vi "NStageMRate Decimation (Host).vi"(11 "multirate filters":T2[](array[typedef])=[{"mMRate_Structure"=enum."FIR", "mMRate_Mode"=2, "mMRate_Factor"=10, "mMRate_FIRParams"={"mMRate_FIR_H"=[0.00020851805806128276, 0.000613272420690698, 0.0014304185003561158, 0.0028435740310915566, 0.005060843192894627, 0.008276672977011198, 0.01263671879692099, 0.018200819196418323, 0.024910685996005263, 0.03256926849828543, 0.040837119060937545, 0.049249902078079846, 0.0572560861411628, 0.06427222716854132, 0.06974798706333393, 0.07323191327535455, 0.07442764407493105, 0.07323191327535455, 0.06974798706333393, 0.06427222716854132, 0.0572560861411628, 0.049249902078079846, 0.040837119060937545, 0.03256926849828543, 0.024910685996005263, 0.018200819196418323, 0.01263671879692099, 0.008276672977011198, 0.005060843192894627, 0.0028435740310915566, 0.0014304185003561158, 0.000613272420690698, 0.00020851805806128276], "mMRate_FIR_IsNyquist?"=FALSE, "mMRate_FIR_IsSymmetric?"=FALSE}, "mMRate_CICParams"={"mMRate_CIC_#Stage"=0, "mMRate_CIC_Lag"=0, "mMRate_CIC_Type"=enum."Lowpass"}, "mMRate_Order"=32, "mMRate_Version"="2.0", "mMRate_Comments"="", "mMRate_RationalFactor"={"mMRate_L"=-1, "mMRate_M"=-1}, "mMRate_Fs"=100000.0, "mMRate_Quantized?"=TRUE, "mMRate_QFilterGain"=1.0, "mMRate_CoefWl"=16, "mMRate_Scaling"={"mMRate_ScaleByPowerOf2?"=TRUE, "mMRate_ScaleType"=enum."Time Domain 1-Norm"}, "mMRate_InputWl"=16, "mMRate_OutputWl"=32, "mMRate_OutputMode"=enum."Nearest", "mMRate_MultMode"=enum."Truncated", "mMRate_BitPruning"=TRUE, "mMRate_GainWl"=-1, "mMRate_OutputFwl"=-30, "mMRate_SumIwl"=2, "mMRate_InputIwl "=1, "mMRate_SumWl"=32, "mMRate_CoefIwl"=0}, {"mMRate_Structure"=enum."FIR", "mMRate_Mode"=2, "mMRate_Factor"=5, "mMRate_FIRParams"={"mMRate_FIR_H"=[-0.0004681667078035737, -0.001767925193669993, -0.003970356160230413, -0.005978286856899856, -0.005090123043269885, 0.0025917170420743487, 0.020602728875030812, 0.04989465476912974, 0.08711166887294974, 0.12459826753370787, 0.15261700974431505, 0.1630150884241493, 0.15261700974431505, 0.12459826753370787, 0.08711166887294974, 0.04989465476912974, 0.020602728875030812, 0.0025917170420743487, -0.005090123043269885, -0.005978286856899856, -0.003970356160230413, -0.001767925193669993, -0.0004681667078035737], "mMRate_FIR_IsNyquist?"=FALSE, "mMRate_FIR_IsSymmetric?"=FALSE}, "mMRate_CICParams"={"mMRate_CIC_#Stage"=0, "mMRate_CIC_Lag"=0, "mMRate_CIC_Type"=enum."Lowpass"}, "mMRate_Order"=22, "mMRate_Version"="2.0", "mMRate_Comments"="", "mMRate_RationalFactor"={"mMRate_L"=-1, "mMRate_M"=-1}, "mMRate_Fs"=10000.0, "mMRate_Quantized?"=TRUE, "mMRate_QFilterGain"=2.0, "mMRate_CoefWl"=16, "mMRate_Scaling"={"mMRate_ScaleByPowerOf2?"=TRUE, "mMRate_ScaleType"=enum."Time Domain 1-Norm"}, "mMRate_InputWl"=32, "mMRate_OutputWl"=32, "mMRate_OutputMode"=enum."Nearest", "mMRate_MultMode"=enum."Truncated", "mMRate_BitPruning"=TRUE, "mMRate_GainWl"=-1, "mMRate_OutputFwl"=-30, "mMRate_SumIwl"=2, "mMRate_InputIwl "=1, "mMRate_SumWl"=32, "mMRate_CoefIwl"=0}, {"mMRate_Structure"=enum."FIR", "mMRate_Mode"=2, "mMRate_Factor"=2, "mMRate_FIRParams"={"mMRate_FIR_H"=[0.00011146621958819476, 0.0002565535621370625, 0.0004667088173512661, 0.0007398841585625596, 0.0009920839582570331, 0.0011689556532843148, 0.0011441466836693446, 0.0008511401604360608, 0.00021389293056072765, -0.0007249166118789748, -0.001870429374643854, -0.002986975146976202, -0.003801687060362348, -0.00398217847599286, -0.0032847785470121646, -0.0015737370213748415, 0.001039829337909637, 0.004217142878609337, 0.007348102949246268, 0.009683947675627079, 0.010426026453898712, 0.00895714640162184, 0.0049852319631378695, -0.001256028389914612, -0.008971566877318085, -0.01679505790083628, -0.022982247471379617, -0.025636735420535735, -0.023082337210652882, -0.014175800343177341, 0.001366955164663819, 0.022832828266504384, 0.04847501833410211, 0.07572360544515389, 0.10149685808514643, 0.12268476783744374, 0.13660407501114266, 0.14145839621127393, 0.13660407501114266, 0.12268476783744374, 0.10149685808514643, 0.07572360544515389, 0.04847501833410211, 0.022832828266504384, 0.001366955164663819, -0.014175800343177341, -0.023082337210652882, -0.025636735420535735, -0.022982247471379617, -0.01679505790083628, -0.008971566877318085, -0.001256028389914612, 0.0049852319631378695, 0.00895714640162184, 0.010426026453898712, 0.009683947675627079, 0.007348102949246268, 0.004217142878609337, 0.001039829337909637, -0.0015737370213748415, -0.0032847785470121646, -0.00398217847599286, -0.003801687060362348, -0.002986975146976202, -0.001870429374643854, -0.0007249166118789748, 0.00021389293056072765, 0.0008511401604360608, 0.0011441466836693446, 0.0011689556532843148, 0.0009920839582570331, 0.0007398841585625596, 0.0004667088173512661, 0.0002565535621370625, 0.00011146621958819476], "mMRate_FIR_IsNyquist?"=FALSE, "mMRate_FIR_IsSymmetric?"=FALSE}, "mMRate_CICParams"={"mMRate_CIC_#Stage"=0, "mMRate_CIC_Lag"=0, "mMRate_CIC_Type"=enum."Lowpass"}, "mMRate_Order"=74, "mMRate_Version"="2.0", "mMRate_Comments"="", "mMRate_RationalFactor"={"mMRate_L"=-1, "mMRate_M"=-1}, "mMRate_Fs"=2000.0, "mMRate_Quantized?"=TRUE, "mMRate_QFilterGain"=2.0, "mMRate_CoefWl"=16, "mMRate_Scaling"={"mMRate_ScaleByPowerOf2?"=TRUE, "mMRate_ScaleType"=enum."Time Domain 1-Norm"}, "mMRate_InputWl"=32, "mMRate_OutputWl"=16, "mMRate_OutputMode"=enum."Nearest", "mMRate_MultMode"=enum."Truncated", "mMRate_BitPruning"=TRUE, "mMRate_GainWl"=-1, "mMRate_OutputFwl"=-14, "mMRate_SumIwl"=2, "mMRate_InputIwl "=1, "mMRate_SumWl"=32, "mMRate_CoefIwl"=0}] {"mMRate_SumWl" min=1 max=32 step=1; "mMRate_InputIwl" min=1 max=32 step=1; "mMRate_GainWl" min=1 max=32 step=1; "mMRate_OutputWl" min=1 max=32 step=1; "mMRate_InputWl" min=1 max=32 step=1; "mMRate_CoefWl" min=1 max=32 step=1; "mMRate_Mode" items=["Default"=-1, "No Rate Change"=0, "Interpolation"=1, "Decimation"=2, "Interpolated"=3, "Rational"=4]}) -> ()   [LabVIEW 2023]
uses:
  <vilib>/rvi/interface/nirviOpenFPGA/nirviOpenFPGA.xnode
  <vilib>/rvi/interface/nirviMethod/nirviMethod.xnode
  <vilib>/addons/Digital Filter Design/NI_DigFilterLicensed.lvlib
  <vilib>/addons/Digital Filter Design/FXPMRateSim.llb/DFD FXP NStage MRate Postprocessing (I32, nCh).vi
  <vilib>/rvi/interface/nirviCloseFPGA/nirviCloseFPGA.xnode
  <vilib>/rvi/errors/niLvFpgaMergeErrorWithErrorCode.vi
  FPGA Bitfiles/NStageMRateDecim_DFDTFilterTarget_NStageMRateDecim_u6L7F1v0Zk0.lvbitx
  NStageMRate Decimation (FPGA).vi
  <vilib>/addons/Digital Filter Design/_Objects.llb/DFD Multirate Mode.ctl
  <vilib>/addons/Digital Filter Design/_Objects.llb/DFD Coef Norm Type.ctl
  <vilib>/addons/Digital Filter Design/_Objects.llb/DFD FXP MRate Multiply Mode.ctl
  <vilib>/addons/Digital Filter Design/_Objects.llb/DFD Round-off Mode.ctl
  <vilib>/addons/Digital Filter Design/_Objects.llb/DFD Multirate Filter Obj.ctl
  <vilib>/userdefined/High Color/nirio_resource_hc.ctl
panel:
  in  "Resource Name":T1="RIO0::INSTR"
  in  "stop":bool
  out "Filtered Signal":dbl[][](graph)
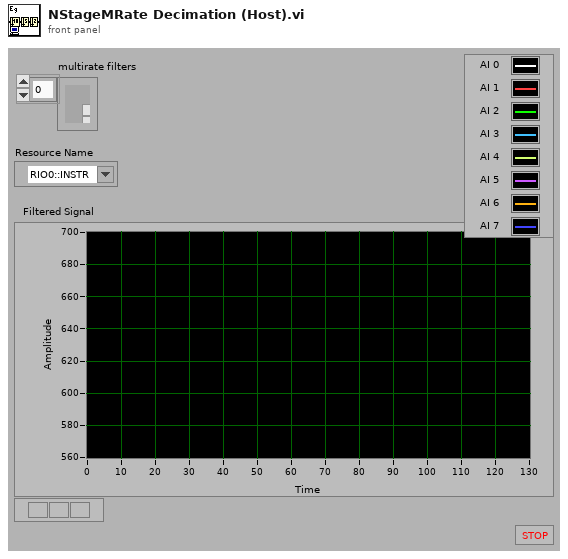
[diagram p1: front panel]
types:
  T1 = typedef "nirio_resource_hc.ctl" = tag
  T2 = typedef "NI_DigFilterLicensed.lvlib/DFD Multirate Filter Obj.ctl" = cluster{"mMRate_Structure":enum16{"CIC", "FIR", "IIR", "Lattice"}, "mMRate_Mode":T3, "mMRate_Factor":i32, "mMRate_FIRParams":cluster{"mMRate_FIR_H":dbl[], "mMRate_FIR_IsNyquist?":bool, "mMRate_FIR_IsSymmetric?":bool}, "mMRate_CICParams":cluster{"mMRate_CIC_#Stage":i32, "mMRate_CIC_Lag":i32, "mMRate_CIC_Type":enum16{"Lowpass", "Highpass"}}, "mMRate_Order":i32, "mMRate_Version":string, "mMRate_Comments":string, "mMRate_RationalFactor":cluster{"mMRate_L":i32, "mMRate_M":i32}, "mMRate_Fs":dbl, "mMRate_Quantized?":bool, "mMRate_QFilterGain":dbl, "mMRate_CoefWl":i16, "mMRate_Scaling":cluster{"mMRate_ScaleByPowerOf2?":bool, "mMRate_ScaleType":T4}, "mMRate_InputWl":i16, "mMRate_OutputWl":i16, "mMRate_OutputMode":T5, "mMRate_MultMode":T6, "mMRate_BitPruning":bool, "mMRate_GainWl":i16, "mMRate_OutputFwl":i16, "mMRate_SumIwl":i16, "mMRate_InputIwl ":i16, "mMRate_SumWl":i16, "mMRate_CoefIwl":i16}
  T3 = typedef "NI_DigFilterLicensed.lvlib/DFD Multirate Mode.ctl" = i16
  T4 = typedef "NI_DigFilterLicensed.lvlib/DFD Coef Norm Type.ctl" = enum16{"No Norm", "Time Domain 1-Norm", "Time Domain 2-Norm", "Time Domain Inf-Norm"}
  T5 = typedef "NI_DigFilterLicensed.lvlib/DFD Round-off Mode.ctl" = enum16{"Nearest", "Truncation"}
  T6 = typedef "NI_DigFilterLicensed.lvlib/DFD FXP MRate Multiply Mode.ctl" = enum16{"Truncated", "Full"}
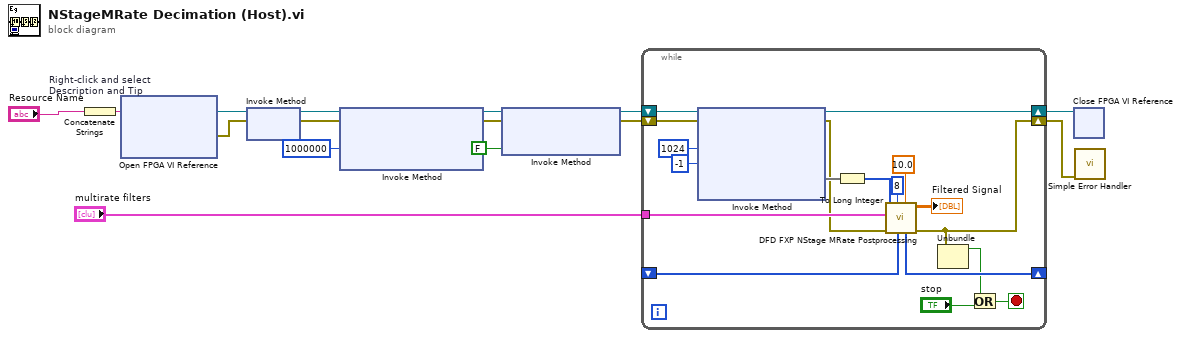
[diagram p0: block diagram]
diagram:
  n1 = Concatenate Strings "Right-click and select Description and Tip"("Resource Name") -> (w1:string)
  n2 = xnode "Open FPGA VI Reference"("resource name"=w1) -> ("FPGA VI Reference Out"=w15:refnum<k20>, "error out"=w14:errorcluster)  [unwired: 1 in]
  n3 = xnode "Invoke Method"("FPGA VI Reference In"=w15, "error in"=w14) -> ("FPGA VI Reference Out"=w13:refnum<k20>, "error out"=w12:errorcluster)
  n4 = xnode "Invoke Method"("FPGA VI Reference In"=w13, "error in"=w12, "Requested Depth"=u32 1000000 ("Depth")) -> ("FPGA VI Reference Out"=w10:refnum<k20>, "error out"=w9:errorcluster)  [unwired: 1 out]
  n5 = xnode "Invoke Method"("FPGA VI Reference In"=w10, "error in"=w9, "Wait Until Done (F)"=FALSE) -> ("FPGA VI Reference Out"=w8:refnum<k20>, "error out"=w7:errorcluster)
  n6 = while {
    shift-right: [w19] -> w4
    shift-left: w7 -> [w32]
    tunnel: "multirate filters" -> [w27]
    shift-right: [w24] -> _
    shift-left: _ -> [w23]
    shift-right: [w20] -> w5
    shift-left: w8 -> [w33]
    stop <- w16 stop-if-true
    n7 = xnode "Invoke Method"("FPGA VI Reference In"=w33, "error in"=w32, "Number of Elements"=u32 1024, "Timeout (ms)"=-1) -> ("FPGA VI Reference Out"=w20:refnum<k20>, "error out"=w25:errorcluster, "Data"=w29:void[])  [unwired: 1 out]
    n8 = To Long Integer(number=w29) -> (32bit integer=w28:i32[])
    n9 = call-poly <vilib>:"DFD FXP NStage MRate Postprocessing.vi"("input range"=10.0, "history in"=w23, "# channels"=8, "error in (no error)"=w25, "multirate filters"=w27, "signal in"=w28) -> ("error out"=w19:errorcluster, "signal out"=→"Filtered Signal":dbl[][], "history out"=w24:i32[])  [unwired: 3 out]
    n10 = Unbundle(w19) -> ("status"=w17:bool)  [unwired: 2 out]
    n11 = Or(x=w17, y="stop") -> (x .or. y?=w16:bool)
  }
  n12 = xnode "Close FPGA VI Reference"("FPGA VI Reference In"=w5) -> ()  [unwired: 1 in, 1 out]
  n13 = call <vilib>:"Simple Error Handler.vi"("error in (no error)"=w4) -> ()  [unwired: 1 in, 8 out]
